vi "Create Pattern Script - Rd Data Compare Frame.vi"(8 "error in (no error)":errorcluster, 11 "BML Pattern Creater in":refnum<class "BML Pattern Creater.lvclass">) -> (0 "error out":errorcluster, 2 "RdDataCompare":string, 3 "BML Pattern Creater out":refnum<class "BML Pattern Creater.lvclass">)   [LabVIEW 2018, in "BML Pattern Creater.lvlib" / "BML Pattern Creater.lvclass"]
uses:
  BML Pattern Creater.lvclass
  C:/P4 Workspace/PC Client/Solutions/5g_eap/trunk/1.0/HiSi5GmmWave/Pattern_Gen_Tool/Interfaces/Protocol Interface.lvlibp/Interfaces/Protocol Interface/Protocol Interface.lvclass
  Ctls/OM - BML.ctl
  BML Pattern Creater.lvclass/BML Pattern Creater.ctl
  Write BML OM.vi
  Read Frame Data.vi
  Interfaces/Protocol Interface.lvlibp/Interfaces/Protocol Interface/Read Num of cycle Rd.vi
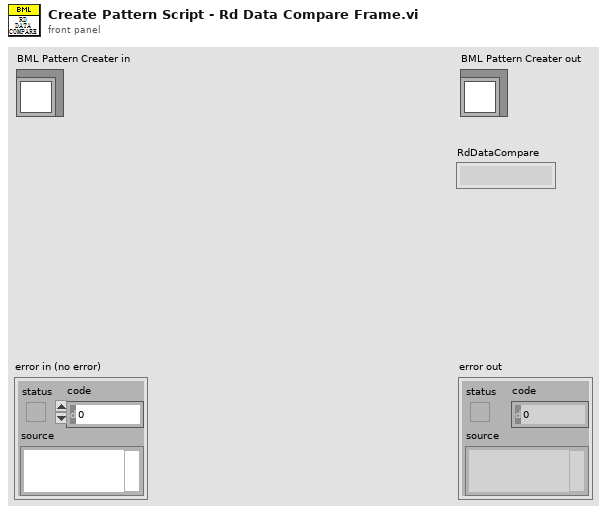
[diagram p1: front panel]
types:
  T1 = typedef "OM - BML.ctl" = enum16{"Normal", "ImmeEffect", "InitSlaveID", "LoadData"}
  T2 = typedef "FRM Data - BML.ctl" = cluster{"Pattern_Name":string, "Data":u8[], "Start_Addr":u16, "ChipID":u8, "num of wait ms":i8, "Opcode":string[], "BML OM":T1, "BurstLength":T3, "FSN":u8, "R/W?":T4}
  T3 = typedef "Burst Length.ctl" = enum8{"0", "2", "3", "4", "5", "8", "16", "32"}
  T4 = typedef "RW Options.ctl" = enum16{"Read", "Write", "R/W"}
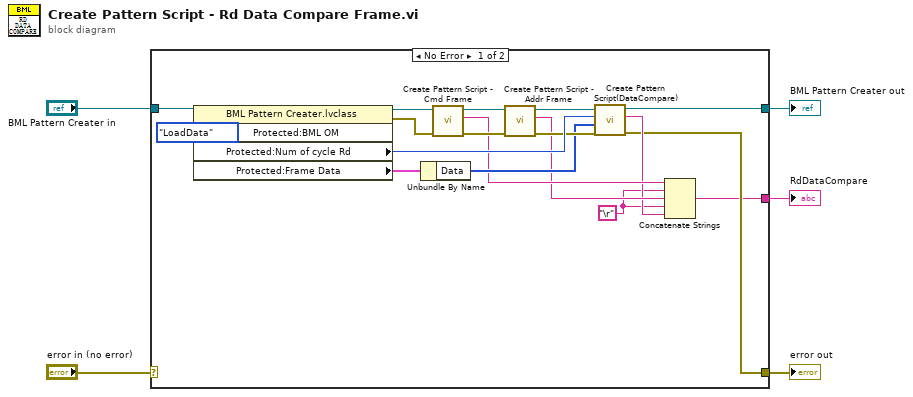
[diagram p0: block diagram]
diagram:
  n1 = case shown="No Error" "error in (no error)" {
    selector: "error in (no error)" -> [_ w25]
    tunnel: [w7 w25] -> w4
    tunnel: [w8 w24] -> w2
    tunnel: "BML Pattern Creater in" -> [w23 w24]
    tunnel: [w6 _] -> w1
    frame No Error {
      w9 = "\r"
      n2 = property class="BML Pattern Creater.lvclass"(reference=w23, "Protected:BML OM"=OM_-_BML."LoadData" ("BML OM")) -> (reference out=w21:refnum<class "BML Pattern Creater.lvclass">, error out=w20:errorcluster, "Protected:Num of cycle Rd"=w16:u32, "Protected:Frame Data"=w14:T2)  [unwired: 1 in]
      n3 = Unbundle By Name(w14) -> ("Data"=w13:u8[])
      n4 = call "Create Pattern Script - Cmd Frame.vi"("error in (no error)"=w20, "BML Pattern Creater in"=w21) -> ("error out"=w18:errorcluster, "CMD Frame out"=w12:string, "BML Pattern Creater out"=w19:refnum<class "BML Pattern Creater.lvclass">)  [unwired: 7 in]
      n5 = call "Create Pattern Script - Addr Frame.vi"("error in (no error)"=w18, "BML Pattern Creater in"=w19) -> ("error out"=w15:errorcluster, "Addr Frame"=w11:string, "BML Pattern Creater out"=w17:refnum<class "BML Pattern Creater.lvclass">)  [unwired: 7 in]
      n6 = call "Create Pattern Script(DataCompare).vi"("error in (no error)"=w15, "Data"=w13, "Num of wait cycle for read"=w16, "BML Pattern Creater in"=w17) -> ("error out"=w7:errorcluster, "String"=w10:string, "BML Pattern Creater out"=w8:refnum<class "BML Pattern Creater.lvclass">)  [unwired: 5 in]
      n7 = Concatenate Strings(w12, w9, w11, w9, w10) -> (w6:string)
    }
    frame Error {
    }
  }
  "error out" <- w4
  "BML Pattern Creater out" <- w2
  "RdDataCompare" <- w1
